vi "保存当时的实时图片 - 副本.vi"(11 "Browser Size":cluster{"X":i32, "Y":i32}) -> (3 "Image Browser Out":T1)   [LabVIEW 2017]
uses:
  <vilib>/vision/Image Controls.llb/IMAQ Image.ctl
  <vilib>/vision/NI_Vision_Development_Module.lvlib
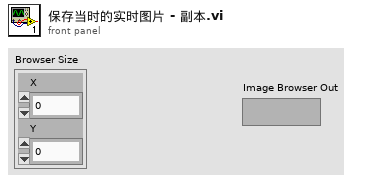
[diagram p1: front panel]
types:
  T1 = typedef "IMAQ Image.ctl" = refnum<image>
  T2 = cluster{"Browser Size":cluster{"X":i32, "Y":i32}, "Images per Line":i32, "Background Color":u32, "Frame Size":i32, "Frame Style":u16}
  T3 = typedef "Image Type" = u32
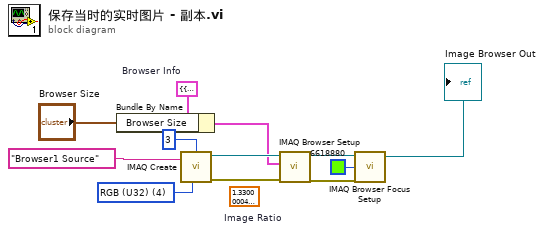
[diagram p0: block diagram]
diagram:
  w5 = T2 {"Browser Size"={"X"=300, "Y"=200}, "Images per Line"=3, "Background Color"=14869218, "Frame Size"=3, "Frame Style"=0}  # Browser Info
  (unwired) sgl 1.33  # Image Ratio
  w10 = T3 4 items=["Grayscale (U8)", "Grayscale (I16)", "Grayscale (SGL)", "Complex (CSG)", "RGB (U32)", "HSL (U32)", "RGB (U64)", "Grayscale (U16)"] ("Image Type")
  n1 = Bundle By Name(cluster=w5, "Browser Size"="Browser Size") -> (w4:T2)
  n2 = call "IMAQ Create"("Border Size"=3, "Image Name"="Browser1 Source", "Image Type"=w10) -> ("New Image"=w12:T1, "error out"=w11:errorcluster)  [unwired: 2 in]
  n3 = call "IMAQ Browser Setup"("error in (no error)"=w11, "Browser Info"=w4, "Image In"=w12) -> ("error out"=w7:errorcluster, "Image Browser Out"=w8:T1)  [unwired: 1 in, 2 out]
  n4 = call "IMAQ Browser Focus Setup"("error in (no error)"=w7, "Focus Color"=u32 6618880, "Image Browser In"=w8) -> ("Image Browser Out"=→"Image Browser Out":T1)  [unwired: 1 in, 1 out]
